vi "Write Truth Table.vi"(10 "Truth Table":T1(array[cluster]), 11 "Maxscend SP4T in":refnum<class "Maxscend SP4T.lvclass">) -> (3 "Maxscend SP4T out":refnum<class "Maxscend SP4T.lvclass">)   [LabVIEW 2020, in "Maxscend SP4T.lvclass"]
uses:
  Maxscend SP4T.lvclass
  Maxscend SP4T.lvclass/Maxscend SP4T.ctl
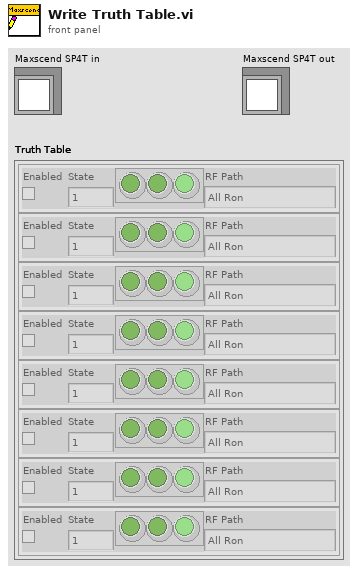
[diagram p1: front panel]
types:
  T1 = cluster{"Enabled":bool, "State":dbl, "V1 V2 V3":bool[], "RF Path":string}[]
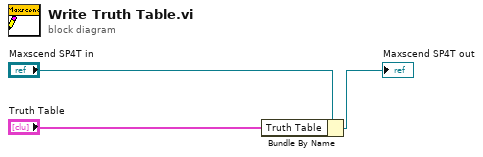
[diagram p0: block diagram]
diagram:
  n1 = Bundle By Name(cluster="Maxscend SP4T in", "Truth Table"="Truth Table") -> (→"Maxscend SP4T out":refnum<class "Maxscend SP4T.lvclass">)
